vi "pythontest.vi"() -> ()   [LabVIEW 2019]
panel:
  out "configItem":string
  in  "GUID":string
  out "return value":string
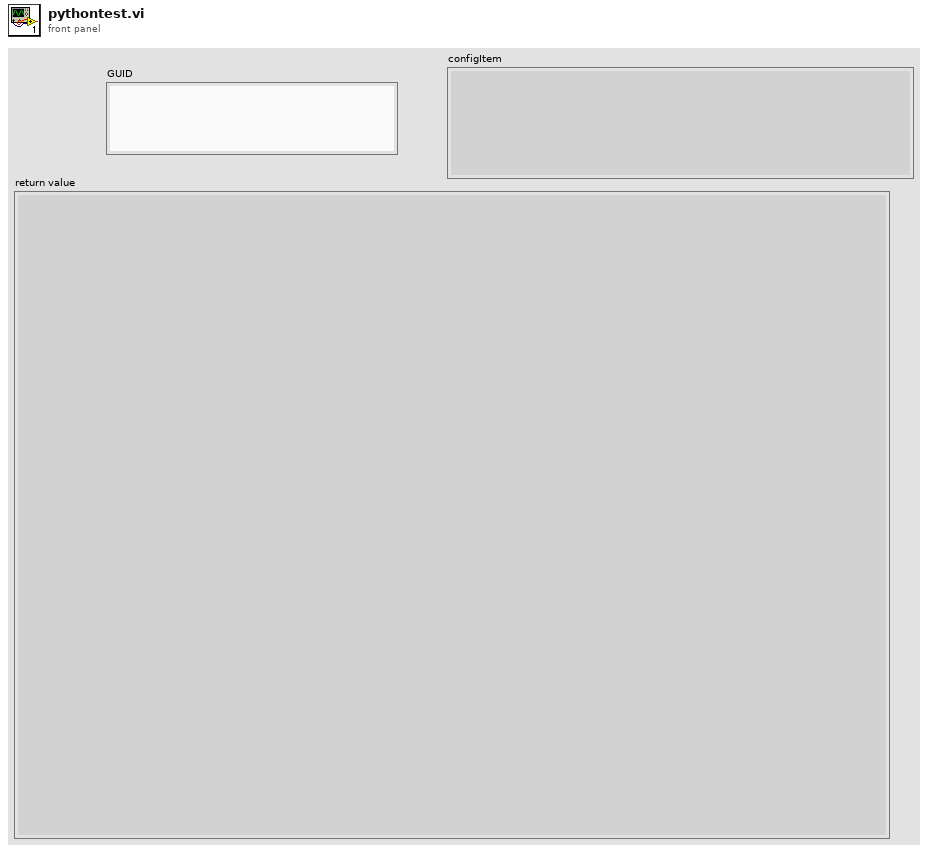
[diagram p1: front panel]
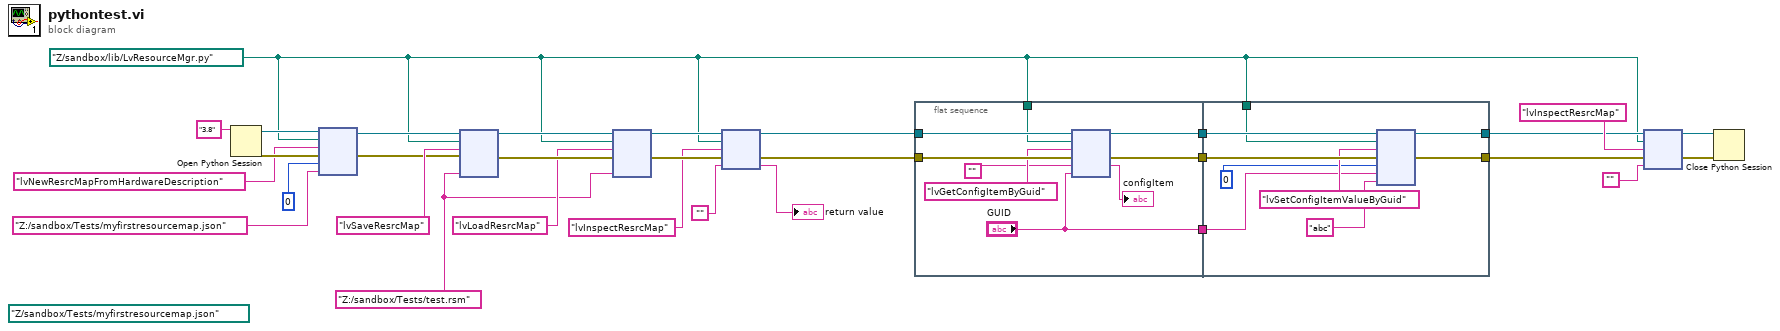
[diagram p0: block diagram]
diagram:
  w18 = "Z:/sandbox/Tests/test.rsm" ("function name")
  (unwired) path "Z:/sandbox/Tests/myfirstresourcemap.json" ("module path")
  w1 = path "Z:/sandbox/lib/LvResourceMgr.py" ("module path")
  n1 = Open Python Session(python version="3.8" ("Python version")) -> (session out=w29:refnum<k35>, error out=w30:errorcluster)  [unwired: 2 in]
  n2 = node(w29, w1, "lvNewResrcMapFromHardwareDescription" ("function name"), w30, 0, "Z:/sandbox/Tests/myfirstresourcemap.json" ("function name")) -> (w24:refnum<k35>, w22:errorcluster)  [unwired: 2 in, 2 out]
  n3 = node(w24, w1, "lvSaveResrcMap" ("function name"), w22, w18) -> (w21:refnum<k35>, w20:errorcluster)  [unwired: 3 in, 2 out]
  n4 = node(w21, w1, "lvLoadResrcMap" ("function name"), w20, w18) -> (w17:refnum<k35>, w16:errorcluster)  [unwired: 3 in, 2 out]
  n5 = node(w17, w1, "lvInspectResrcMap" ("function name"), w16, "") -> (w12:refnum<k35>, w11:errorcluster, →"return value":string)  [unwired: 2 out]
  n6 = flat-sequence {
    tunnel: w12 -> [w39]
    tunnel: w11 -> [w38]
    tunnel: w1 -> [w37]
    tunnel: [w35] -> w10
    tunnel: [w34] -> w9
    tunnel: ["GUID"] -> w8
    tunnel: [w47] -> w4
    tunnel: [w46] -> w5
    tunnel: w10 -> [w45]
    tunnel: w9 -> [w48]
    tunnel: w8 -> [w42]
    tunnel: w1 -> [w44]
    frame #0 {
      n7 = node(w39, w37, "lvGetConfigItemByGuid" ("function name"), w38, "", "GUID") -> (w34:refnum<k35>, w35:errorcluster, →"configItem":string)  [unwired: 1 in, 2 out]
    }
    frame #1 {
      n8 = node(w48, w44, "lvSetConfigItemValueByGuid" ("function name"), w45, 0, w42, "abc") -> (w47:refnum<k35>, w46:errorcluster)  [unwired: 3 in, 2 out]
    }
  }
  n9 = node(w4, w1, "lvInspectResrcMap" ("function name"), w5, "") -> (w2:refnum<k35>, w3:errorcluster)  [unwired: 1 in, 2 out]
  n10 = Close Python Session(session in=w2, error in=w3) -> ()  [unwired: 1 out]
